vi "Bus Interface.vi"(0 "AddressSpace":refnum<class "AddressSpace.lvclass">, 1 "abort":bool, 5 "instruction":T2, 9 "input valid":bool) -> (6 "response":T1, 10 "done":bool, 14 "ready for input":bool)   [LabVIEW 2017, in "ActiveFrontEnd.lvlib" / "AddressSpace.lvclass"]
uses:
  AddressSpace.lvclass
  <instrlib>/_niInstr/Instruction Framework/v1/FPGA/Interfaces/Address Space/Address Space Instruction.ctl
  <instrlib>/_niInstr/Instruction Framework/v1/FPGA/Typedefs/Response.ctl
  AddressSpace.lvclass/AddressSpace.ctl
  <vilib>/Utility/error.llb/Clear Errors.vi
  <vilib>/rvi/Emulation/niFpgaSctlEmulationGetInTimedLoop.vi
  <vilib>/rvi/Emulation/niFpgaProcessEmulError.vi
  <vilib>/rvi/DataTransferAndStorage/Container/Common/niFpgaContainerGetUniqueNameForEmu.vi
  <vilib>/rvi/Memory/Memory_Emulation/nirvimemoryEmulationManagerCache_SetValue.vi
  <vilib>/rvi/Memory/Memory_Emulation/nirvimemoryEmulationManagerCache_GetValue.vi
  <vilib>/rvi/Memory/Memory_Emulation/nirvimemoryEmulationManagerCache_ReleaseExclusive.vi
  <vilib>/rvi/Memory/Memory_Emulation/nirvimemoryEmulationManagerCache_InsertValue.vi
  <vilib>/rvi/Memory/Memory_Emulation/niFpgaMemoryEmulationValidateCache.vi
  <vilib>/rvi/Memory/Memory_Emulation/nirvimemoryEmulationManagerCache_MakeExclusive.vi
  <vilib>/rvi/Memory/Memory_Emulation/niFpgaMemoryEmulationCacheClearOnFirstRun.vi
  <vilib>/rvi/Emulation/niFpgaEmulationIsFPGAContextNoSignature.vi
  <vilib>/rvi/DataTransferAndStorage/Container/Common/niFpgaContainerExecOnDevCompGetState.vi
  <vilib>/rvi/DataTransferAndStorage/Container/XNode/niFpgaContainer.xnode
  <vilib>/rvi/DataTransferAndStorage/Register/Emulation/niFpgaRegisterEmulationRefIn.vi
  <instrlib>/_niInstr/Instruction Framework/v1/FPGA/Typedefs/niInstr Instruction Framework v1 FPGA.lvlib
  <instrlib>/_niInstr/Instruction Framework/v1/FPGA/Interfaces/Address Space/Address Space.lvclass
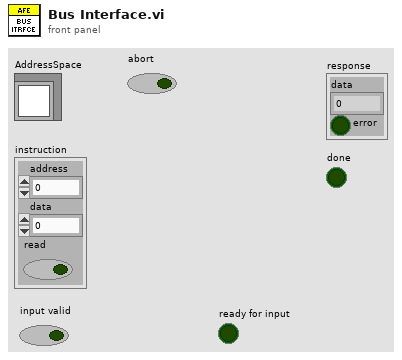
[diagram p1: front panel]
types:
  T1 = typedef "niInstr Instruction Framework v1 FPGA.lvlib/Response.ctl" = cluster{"data":u64, "error":bool}
  T2 = typedef "niInstr Instruction Framework Interfaces v1 FPGA.lvlib/Address Space.lvclass/Address Space Instruction.ctl" = cluster{"address":u32, "data":u64, "read":bool}
  T3 = cluster{"VDCLink_setpt":sgl, "VDCLinkRampRate":sgl, "Q_setpt":sgl, "Pf_setpt":sgl, "Mode":enum16{"Q Control", "Pf Control"}, "perturbance_amp":sgl, "perturbance_freq":sgl, "dT":sgl}
  T4 = cluster{"gains":cluster{"proportional gain":sgl, "integral gain":sgl}, "output range":cluster{"output high (Inf)":sgl, "output low (-Inf)":sgl}, "PI_state":enum8{"idle", "normal", "manual", "perturbance"}, "reset":bool, "manual":sgl}
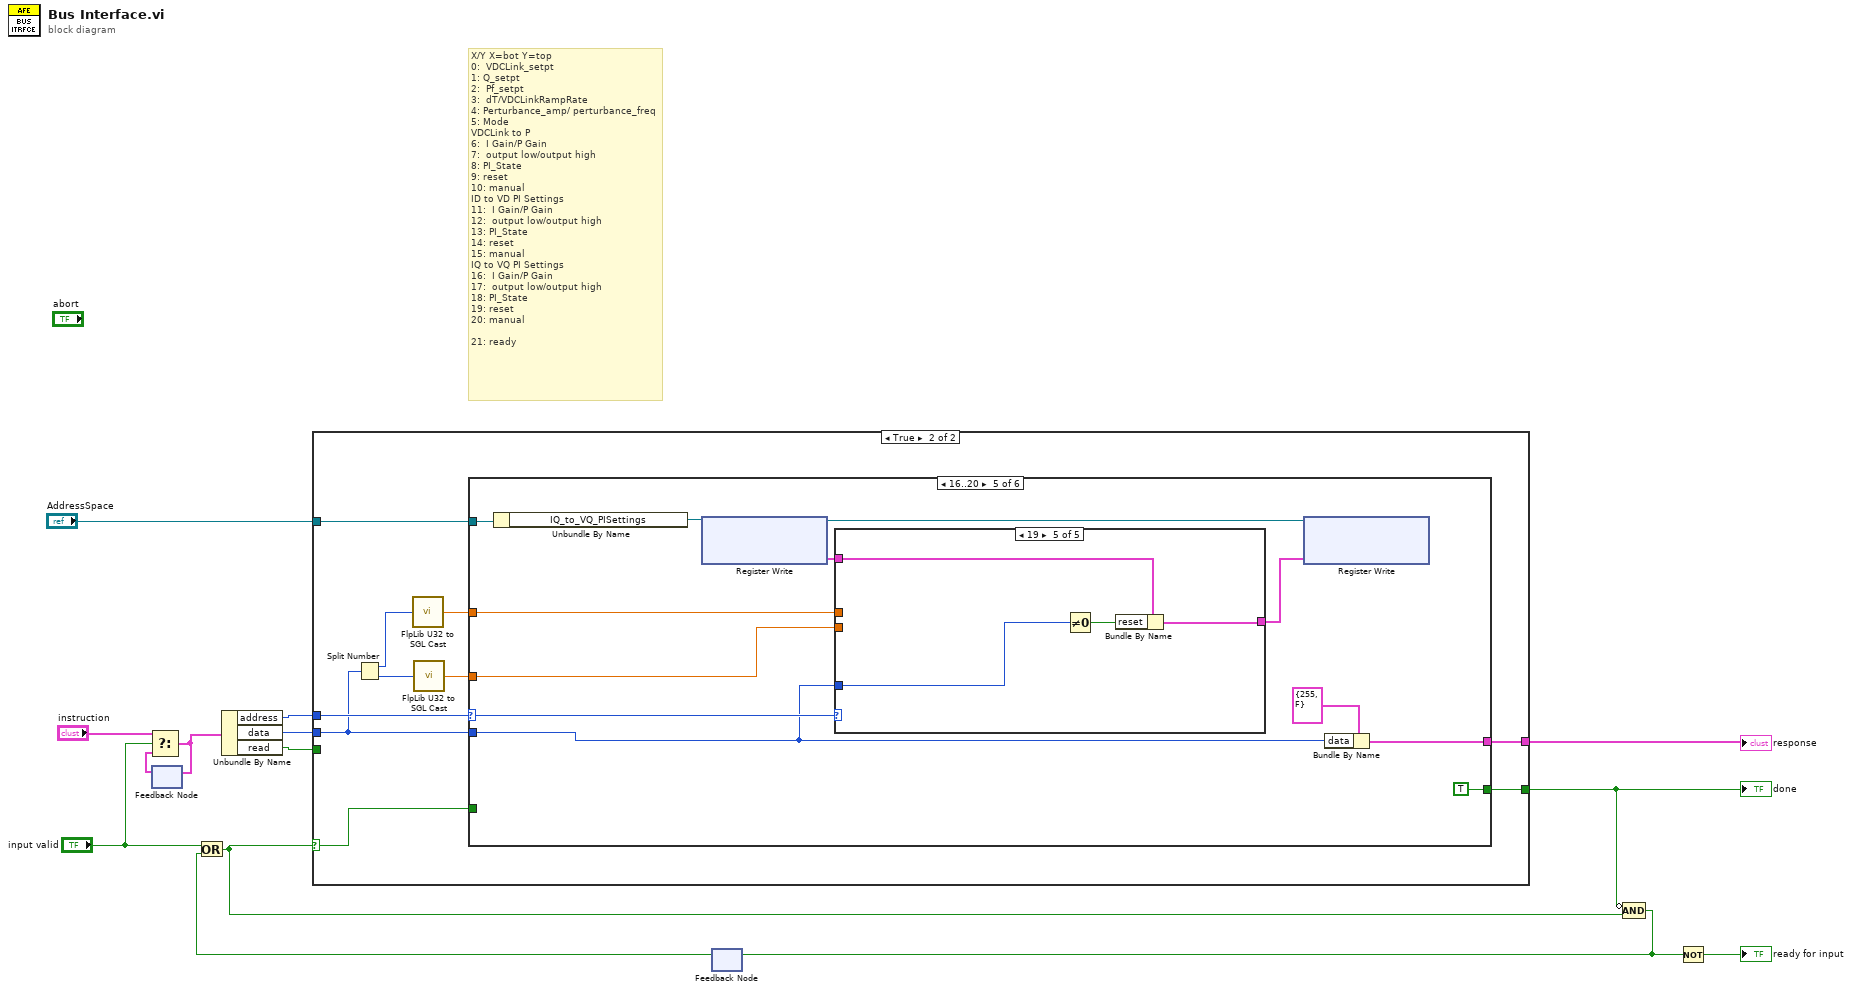
[diagram p0: block diagram]
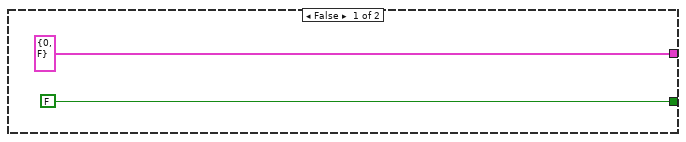
[diagram p2: hidden frame]
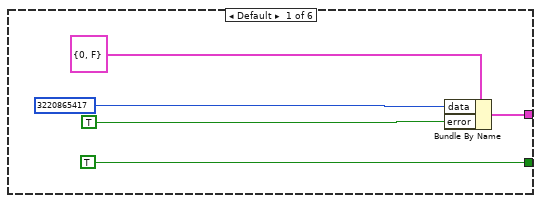
[diagram p3: hidden frame]
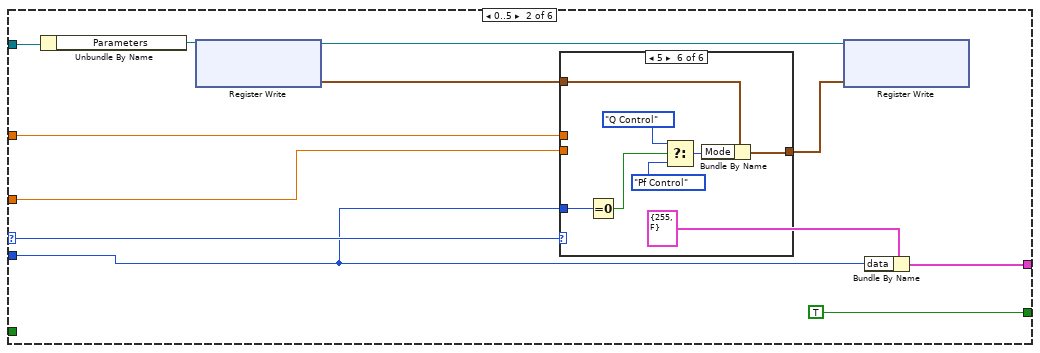
[diagram p4: hidden frame]
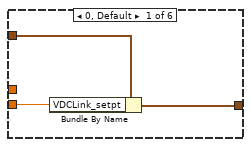
[diagram p5: hidden frame]
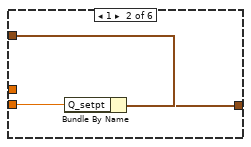
[diagram p6: hidden frame]
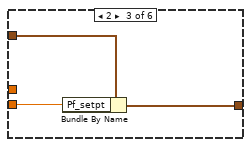
[diagram p7: hidden frame]
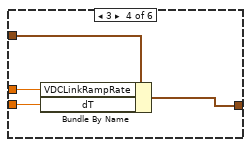
[diagram p8: hidden frame]
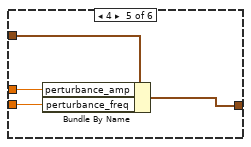
[diagram p9: hidden frame]
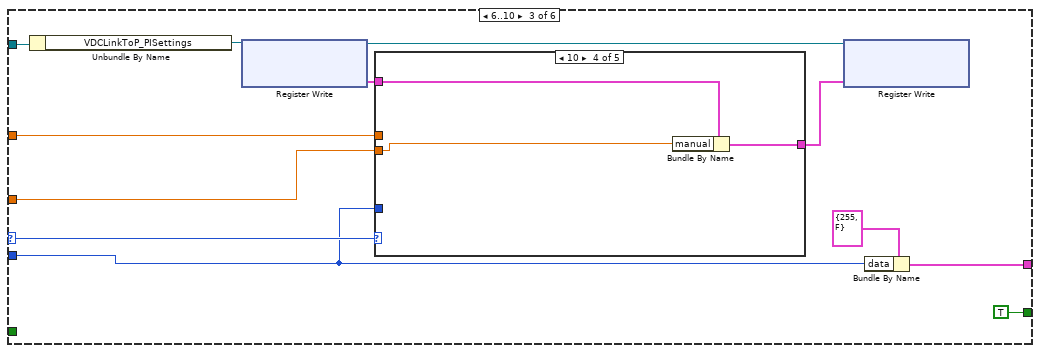
[diagram p10: hidden frame]
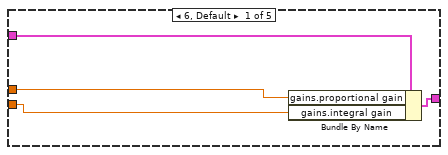
[diagram p11: hidden frame]
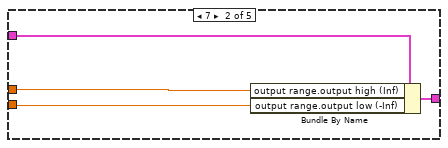
[diagram p12: hidden frame]
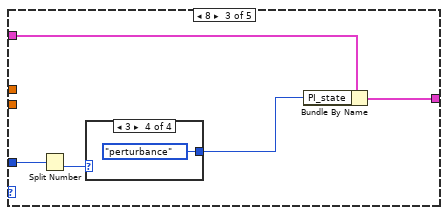
[diagram p13: hidden frame]
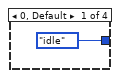
[diagram p14: hidden frame]
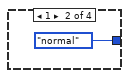
[diagram p15: hidden frame]
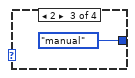
[diagram p16: hidden frame]
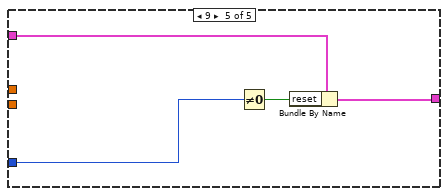
[diagram p17: hidden frame]
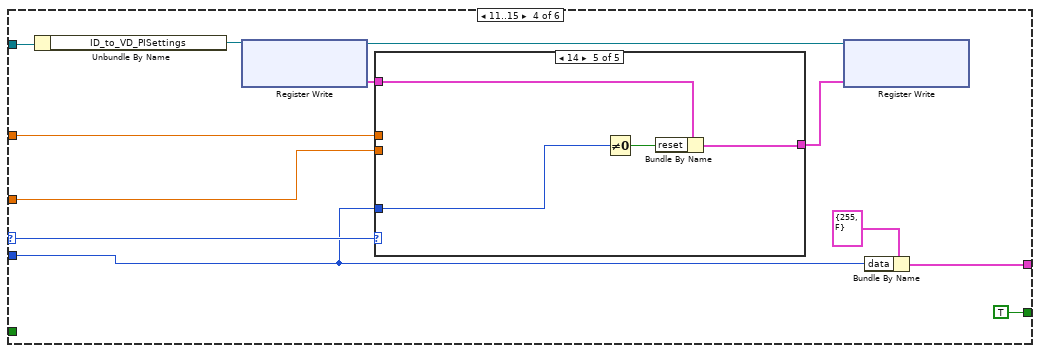
[diagram p18: hidden frame]
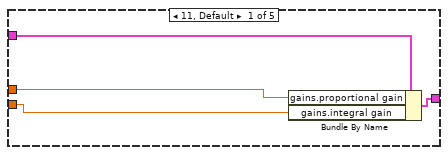
[diagram p19: hidden frame]
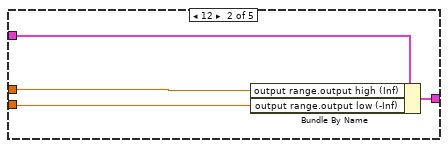
[diagram p20: hidden frame]
diagram:
  # "X/Y X=bot Y=top\n0:  VDCLink_setpt\n1: Q_setpt\n2:  Pf_setpt\n3:  dT/VDCLinkRampRate\n4: Perturbance_amp/ perturbance_freq\n5: Mode\nVDCLink to P\n6:  I Gain/P Gain\n7:  output low/output high\n8: PI_State\n9: reset\n10: manual\nID to VD PI Settings \n11:  I Gain/P Gain\n12:  output low/output high\n13: PI_State\n14: reset\n15: manual\nIQ to VQ PI Settings\n16:  I Gain/P Gain\n17:  output low/output high\n18: PI_State\n19: reset\n20: manual\n\n21: ready"
  n1 = feedback #1() -> (w14:T2)  [unwired: 1 in]
  n2 = Select(t="instruction", s="input valid", f=w14) -> (s? t:f=w13:T2)
  n3 = feedback-in #1(w13) -> ()
  n4 = Unbundle By Name(w13) -> ("address"=w10:u32, "data"=w11:u64, "read"=w12:bool)
  n5 = feedback #2() -> (w7:bool)  [unwired: 1 in]
  n6 = Or(x="input valid", y=w7) -> (x .or. y?=w8:bool)
  n7 = case shown="True" w8 {
    selector: w8 -> [_ w22]
    tunnel: w12 -> [_ _]
    tunnel: w10 -> [_ w26]
    tunnel: w11 -> [_ w21]
    tunnel: [T1 {"data"=0, "error"=FALSE} ("response") w25] -> w5
    tunnel: [FALSE ("Output Valid") w24] -> w4
    tunnel: "AddressSpace" -> [_ w23]
    frame False {
    }
    frame True {
      n8 = Split Number(x=w21) -> (hi(x)=w18:u32, lo(x)=w20:u32)
      n9 = call <userlib>:"FlpLib U32 to SGL Cast.vi"("x"=w18) -> ("y"=w17:sgl)  [unwired: 4 in]
      n10 = call <userlib>:"FlpLib U32 to SGL Cast.vi"("x"=w20) -> ("y"=w19:sgl)  [unwired: 4 in]
      n11 = case shown="16..20" w26 {
        selector: w26 -> [_ w35 w71 w107 w143 _]
        tunnel: w21 -> [_ w32 w68 w104 w140 w177]
        tunnel: [w28 w40 w76 w112 w148 w179] -> w25
        tunnel: [TRUE ("done") TRUE ("done") TRUE ("done") TRUE ("done") TRUE ("done") TRUE ("done")] -> w24
        tunnel: w23 -> [_ w43 w79 w115 w151 w182]
        tunnel: w22 -> [_ _ _ _ _ _]
        tunnel: w19 -> [_ w33 w69 w105 w141 _]
        tunnel: w17 -> [_ w34 w70 w106 w142 _]
        frame Default {
          n12 = Bundle By Name(cluster=T1 {"data"=0, "error"=FALSE} ("response"), "data"=u64 3220865417, "error"=TRUE) -> (w28:T1)
        }
        frame 0..5 {
          n13 = Unbundle By Name(w43) -> ("Parameters"=w39:refnum<k21>)
          n14 = xnode ("Register Write")("Register In"=w39) -> ("Data"=w37:T3, "Register Out"=w38:refnum<k21>)
          n15 = case shown="5" w35 {
            tunnel: w37 -> [w46 w49 w52 w56 w60 w67]
            tunnel: [w45 w48 w51 w55 w59 w66] -> w36
            tunnel: w34 -> [_ _ _ w54 w58 _]
            tunnel: w33 -> [w44 w47 w50 w53 w57 _]
            tunnel: w32 -> [_ _ _ _ _ w65]
            frame 0, Default {
              n16 = Bundle By Name(cluster=w46, "VDCLink_setpt"=w44) -> (w45:T3)
            }
            frame 1 {
              n17 = Bundle By Name(cluster=w49, "Q_setpt"=w47) -> (w48:T3)
            }
            frame 2 {
              n18 = Bundle By Name(cluster=w52, "Pf_setpt"=w50) -> (w51:T3)
            }
            frame 3 {
              n19 = Bundle By Name(cluster=w56, "VDCLinkRampRate"=w54, "dT"=w53) -> (w55:T3)
            }
            frame 4 {
              n20 = Bundle By Name(cluster=w60, "perturbance_amp"=w58, "perturbance_freq"=w57) -> (w59:T3)
            }
            frame 5 {
              n21 = Equal To 0?(x=w65) -> (x = 0?=w63:bool)
              n22 = Select(t=enum16{"Q Control", "Pf Control"}."Q Control" ("Mode"), s=w63, f=enum16{"Q Control", "Pf Control"}."Pf Control" ("Mode")) -> (s? t:f=w61:enum16{"Q Control", "Pf Control"})
              n23 = Bundle By Name(cluster=w67, "Mode"=w61) -> (w66:T3)
            }
          }
          n24 = xnode ("Register Write")("Data"=w36, "Register In"=w38) -> ()  [unwired: 1 out]
          n25 = Bundle By Name(cluster=T1 {"data"=255, "error"=FALSE} ("response"), "data"=w32) -> (w40:T1)
        }
        frame 6..10 {
          n26 = Unbundle By Name(w79) -> ("VDCLinkToP_PISettings"=w75:refnum<k21>)
          n27 = xnode ("Register Write")("Register In"=w75) -> ("Data"=w73:T4, "Register Out"=w74:refnum<k21>)
          n28 = case shown="10" w71 {
            tunnel: w73 -> [w83 w87 w92 w99 w103]
            tunnel: [w82 w86 w91 w98 w102] -> w72
            tunnel: w70 -> [w81 w85 _ _ _]
            tunnel: w69 -> [w80 w84 _ w97 _]
            tunnel: w68 -> [_ _ w90 _ w100]
            frame 6, Default {
              n29 = Bundle By Name(cluster=w83, "gains.proportional gain"=w81, "gains.integral gain"=w80) -> (w82:T4)
            }
            frame 7 {
              n30 = Bundle By Name(cluster=w87, "output range.output high (Inf)"=w85, "output range.output low (-Inf)"=w84) -> (w86:T4)
            }
            frame 8 {
              n31 = Split Number(x=w90) -> (lo(x)=w89:u32)  [unwired: 1 out]
              n32 = case shown="3" w89 {
                tunnel: [enum8{"idle", "normal", "manual", "perturbance"}."idle" ("PI_state") enum8{"idle", "normal", "manual", "perturbance"}."normal" ("PI_state") enum8{"idle", "normal", "manual", "perturbance"}."manual" ("PI_state") enum8{"idle", "normal", "manual", "perturbance"}."perturbance" ("PI_state")] -> w88
                frame 0, Default {
                }
                frame 1 {
                }
                frame 2 {
                }
                frame 3 {
                }
              }
              n33 = Bundle By Name(cluster=w92, "PI_state"=w88) -> (w91:T4)
            }
            frame 10 {
              n34 = Bundle By Name(cluster=w99, "manual"=w97) -> (w98:T4)
            }
            frame 9 {
              n35 = Not Equal To 0?(x=w100) -> (x != 0?=w101:bool)
              n36 = Bundle By Name(cluster=w103, "reset"=w101) -> (w102:T4)
            }
          }
          n37 = xnode ("Register Write")("Data"=w72, "Register In"=w74) -> ()  [unwired: 1 out]
          n38 = Bundle By Name(cluster=T1 {"data"=255, "error"=FALSE} ("response"), "data"=w68) -> (w76:T1)
        }
        frame 11..15 {
          n39 = Unbundle By Name(w115) -> ("ID_to_VD_PISettings"=w111:refnum<k21>)
          n40 = xnode ("Register Write")("Register In"=w111) -> ("Data"=w109:T4, "Register Out"=w110:refnum<k21>)
          n41 = case shown="14" w107 {
            tunnel: w109 -> [w119 w123 w128 w135 w139]
            tunnel: [w118 w122 w127 w134 w138] -> w108
            tunnel: w106 -> [w117 w121 _ _ _]
            tunnel: w105 -> [w116 w120 _ w133 _]
            tunnel: w104 -> [_ _ w126 _ w136]
            frame 11, Default {
              n42 = Bundle By Name(cluster=w119, "gains.proportional gain"=w117, "gains.integral gain"=w116) -> (w118:T4)
            }
            frame 12 {
              n43 = Bundle By Name(cluster=w123, "output range.output high (Inf)"=w121, "output range.output low (-Inf)"=w120) -> (w122:T4)
            }
            frame 13 {
              n44 = Split Number(x=w126) -> (lo(x)=w125:u32)  [unwired: 1 out]
              n45 = case shown="3" w125 {
                tunnel: [enum8{"idle", "normal", "manual", "perturbance"}."idle" ("PI_state") enum8{"idle", "normal", "manual", "perturbance"}."normal" ("PI_state") enum8{"idle", "normal", "manual", "perturbance"}."manual" ("PI_state") enum8{"idle", "normal", "manual", "perturbance"}."perturbance" ("PI_state")] -> w124
                frame 0, Default {
                }
                frame 1 {
                }
                frame 2 {
                }
                frame 3 {
                }
              }
              n46 = Bundle By Name(cluster=w128, "PI_state"=w124) -> (w127:T4)
            }
            frame 15 {
              n47 = Bundle By Name(cluster=w135, "manual"=w133) -> (w134:T4)
            }
            frame 14 {
              n48 = Not Equal To 0?(x=w136) -> (x != 0?=w137:bool)
              n49 = Bundle By Name(cluster=w139, "reset"=w137) -> (w138:T4)
            }
          }
          n50 = xnode ("Register Write")("Data"=w108, "Register In"=w110) -> ()  [unwired: 1 out]
          n51 = Bundle By Name(cluster=T1 {"data"=255, "error"=FALSE} ("response"), "data"=w104) -> (w112:T1)
        }
        frame 16..20 {
          n52 = Unbundle By Name(w151) -> ("IQ_to_VQ_PISettings"=w147:refnum<k21>)
          n53 = xnode ("Register Write")("Register In"=w147) -> ("Data"=w145:T4, "Register Out"=w146:refnum<k21>)
          n54 = case shown="19" w143 {
            tunnel: w145 -> [w155 w159 w164 w171 w175]
            tunnel: [w154 w158 w163 w170 w174] -> w144
            tunnel: w142 -> [w153 w157 _ _ _]
            tunnel: w141 -> [w152 w156 _ w169 _]
            tunnel: w140 -> [_ _ w162 _ w172]
            frame 16, Default {
              n55 = Bundle By Name(cluster=w155, "gains.proportional gain"=w153, "gains.integral gain"=w152) -> (w154:T4)
            }
            frame 17 {
              n56 = Bundle By Name(cluster=w159, "output range.output high (Inf)"=w157, "output range.output low (-Inf)"=w156) -> (w158:T4)
            }
            frame 18 {
              n57 = Split Number(x=w162) -> (lo(x)=w161:u32)  [unwired: 1 out]
              n58 = case shown="3" w161 {
                tunnel: [enum8{"idle", "normal", "manual", "perturbance"}."idle" ("PI_state") enum8{"idle", "normal", "manual", "perturbance"}."normal" ("PI_state") enum8{"idle", "normal", "manual", "perturbance"}."manual" ("PI_state") enum8{"idle", "normal", "manual", "perturbance"}."perturbance" ("PI_state")] -> w160
                frame 0, Default {
                }
                frame 1 {
                }
                frame 2 {
                }
                frame 3 {
                }
              }
              n59 = Bundle By Name(cluster=w164, "PI_state"=w160) -> (w163:T4)
            }
            frame 20 {
              n60 = Bundle By Name(cluster=w171, "manual"=w169) -> (w170:T4)
            }
            frame 19 {
              n61 = Not Equal To 0?(x=w172) -> (x != 0?=w173:bool)
              n62 = Bundle By Name(cluster=w175, "reset"=w173) -> (w174:T4)
            }
          }
          n63 = xnode ("Register Write")("Data"=w144, "Register In"=w146) -> ()  [unwired: 1 out]
          n64 = Bundle By Name(cluster=T1 {"data"=255, "error"=FALSE} ("response"), "data"=w140) -> (w148:T1)
        }
        frame 21 {
          n65 = Unbundle By Name(w182) -> ("ready"=w178:refnum<k21>)
          n66 = Not Equal To 0?(x=w177) -> (x != 0?=w176:bool)
          n67 = xnode ("Register Write")("Data"=w176, "Register In"=w178) -> ()  [unwired: 1 out]
          n68 = Bundle By Name(cluster=T1 {"data"=255, "error"=FALSE} ("response"), "data"=w177) -> (w179:T1)
        }
      }
    }
  }
  "done" <- w4
  "response" <- w5
  n69 = Compound Arithmetic op=AND(invert w4, w8) -> (w9:bool)
  n70 = feedback-in #2(w9) -> ()
  n71 = Not(x=w9) -> (.not. x?=→"ready for input":bool)
